vi "VisionMeat.vi"() -> ()   [LabVIEW 2011]
uses:
  <vilib>/vision/NI_Vision_Development_Module.lvlib
  Global 1.vi
panel:
  in  "Camera Type":enum16{"206", "1011"}(ring)
  in  "Score Limits":T1={"Rect Coverage"=76.0, "Aspect Ratio"=70.0, "X Edge Strength"=40.0, "Y Edge Strength"=60.0}
  in  "Area Size Limit":i32=444
  in  "Particle Count Limit":i32=10
  out "Target Info":T2(array[cluster])
  in  "Processing":enum32{"Color", "Intensity", "Intensity Open"}(tab)
  in  "Luminance":i32=255
  in  "Saturation":i32=255
  in  "Hue":i32(knob)=65 scale=0.0..255.0
  in  "Margins":cluster{"Hue":i32, "Sat":i32, "Lum":i32}={"Hue"=9, "Sat"=40, "Lum"=19} {"Sat" scale=0.0..40.0; "Lum" scale=0.0..40.0; "Hue" scale=0.0..40.0}
  in  "Range":cluster{"Lower value":sgl, "Upper value":sgl}={"Lower value"=150.0, "Upper value"=255.0} {"Lower value" scale=0.0..255.0; "Upper value" scale=0.0..255.0}
  in  "Range 2":cluster{"Lower value":sgl, "Upper value":sgl}={"Lower value"=150.0, "Upper value"=255.0} {"Lower value" scale=0.0..255.0; "Upper value" scale=0.0..255.0}
  in  "Annotate":bool=TRUE
  out "Original Image":T3(plugin-control)
  out "Processed Image":T3(plugin-control)
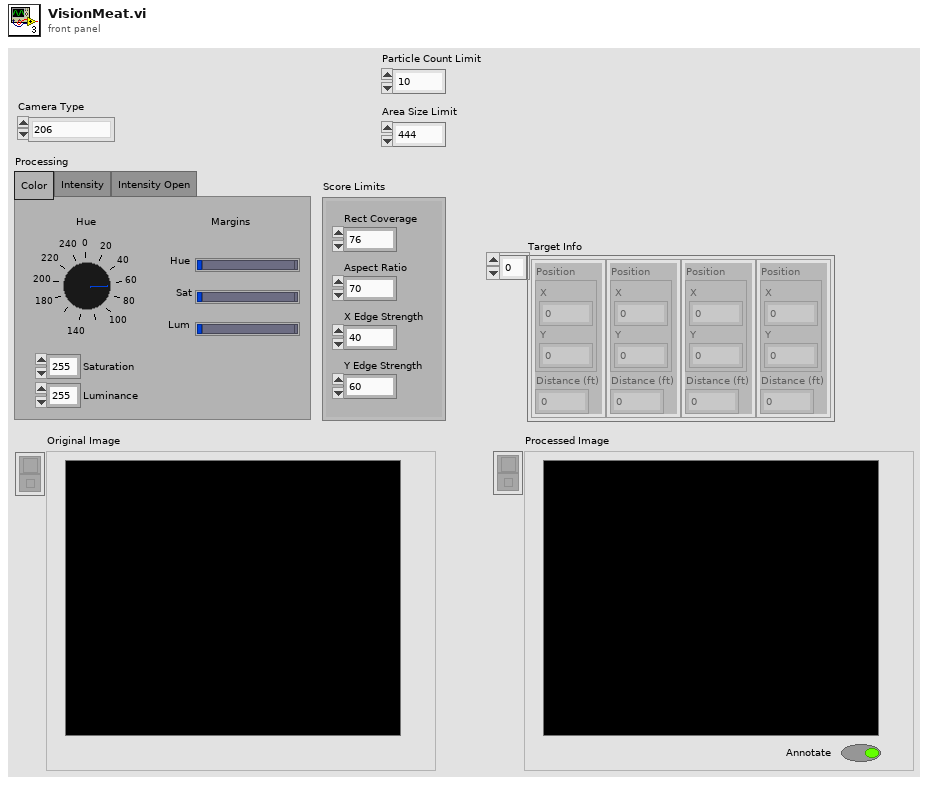
[diagram p1: front panel]
types:
  T1 = cluster{"Rect Coverage":dbl, "Aspect Ratio":dbl, "X Edge Strength":dbl, "Y Edge Strength":dbl}
  T2 = cluster{"Position":cluster{"X":dbl, "Y":dbl}, "Distance (ft)":dbl}[]
  T3 = typedef "IMAQ Image.ctl" = refnum<image>
  T4 = enum32{"AutoM", "Close", "Dilate", "Erode", "Gradient", "Gradient out", "Gradient in", "Hit miss", "Open", "PClose", "POpen", "Thick", "Thin"}
  T5 = cluster{cluster{"Left":dbl, "Top":dbl, "Right":dbl, "Bottom":dbl}, dbl[]}[]
  T6 = cluster{"Left":dbl, "Top":dbl, "Right":dbl, "Bottom":dbl}
  T7 = cluster{"Target Center (-1 to 1)":cluster{"X":dbl, "Y":dbl}, "Distance (ft)":dbl}
  T8 = cluster{"Target Center (-1 to 1)":cluster{"X":dbl, "Y":dbl}, "Distance (ft)":dbl}[]
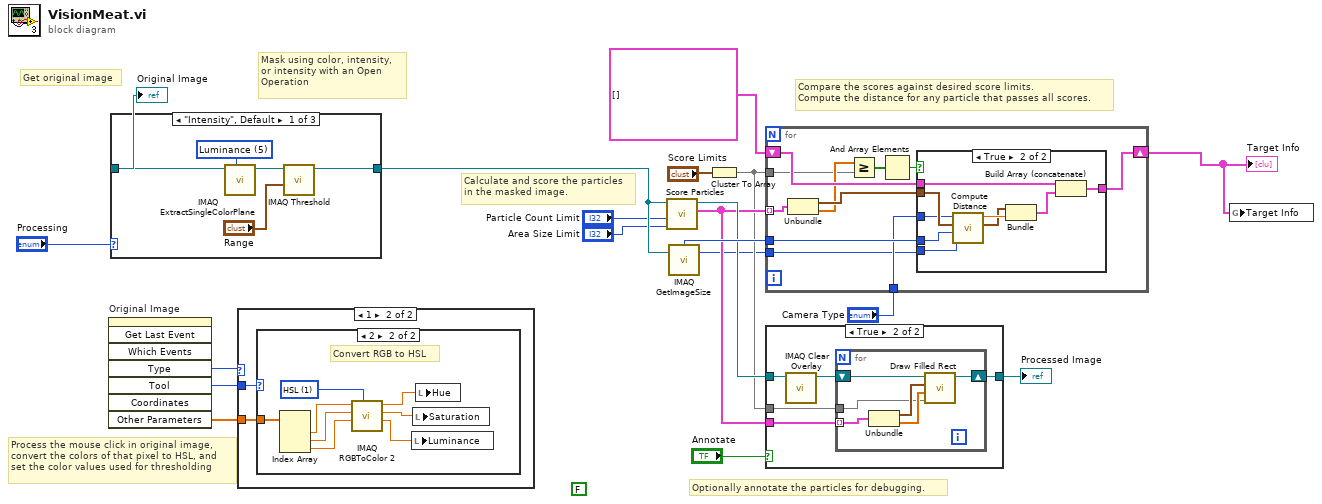
[diagram p0: block diagram]
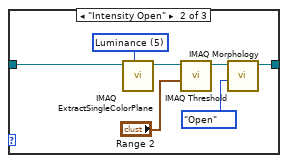
[diagram p3: hidden frame]
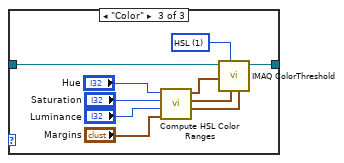
[diagram p4: hidden frame]
diagram:
  (unwired) FALSE
  # "Optionally annotate the particles for debugging."
  # "Compare the scores against desired score limits.\nCompute the distance for any particle that passes all scores."
  # "Process the mouse click in original image,\nconvert the colors of that pixel to HSL, and\nset the color values used for thresholding"
  # "Calculate and score the particles\nin the masked image."
  # "Mask using color, intensity,\nor intensity with an Open\nOperation"
  # "Get original image"
  n1 = invoke on="Original Image" class="ImageControl" method="Get Last Event"() -> ("Type"=w16:i32, "Tool"=w17:i32, "Other Parameters"=w18:sgl[])  [unwired: 8 in, 5 out]
  n2 = case shown="\"Intensity\", Default" "Processing" {
    tunnel: "Original Image" -> [w24 w31 w41]
    tunnel: [w21 w26 w40] -> w7
    frame "Intensity", Default {
      w20 = 5 items=["Red", "Green", "Blue", "Hue", "Saturation", "Luminance", "Value", "Intensity"] ("Color Plane")
      n3 = call "IMAQ ExtractSingleColorPlane"("Color Plane"=w20, "Image Src"=w24) -> ("Image Dst Out"=w23:T3)  [unwired: 2 in, 7 out]
      n4 = call "IMAQ Threshold"("Range"="Range", "Image Src"=w23) -> ("Image Dst Out"=w21:T3)  [unwired: 4 in, 5 out]
    }
    frame "Intensity Open" {
      w25 = 5 items=["Red", "Green", "Blue", "Hue", "Saturation", "Luminance", "Value", "Intensity"] ("Color Plane")
      n5 = call "IMAQ ExtractSingleColorPlane"("Color Plane"=w25, "Image Src"=w31) -> ("Image Dst Out"=w30:T3)  [unwired: 2 in, 7 out]
      n6 = call "IMAQ Threshold"("Range"="Range 2", "Image Src"=w30) -> ("Image Dst Out"=w27:T3)  [unwired: 4 in, 5 out]
      n7 = call "IMAQ Morphology"("Operation"=T4."Open", "Image Src"=w27) -> ("Image Dst Out"=w26:T3)  [unwired: 8 in, 1 out]
    }
    frame "Color" {
      w39 = u16 1 items=["RGB", "HSL", "HSV", "HSI"] ("Color Mode")
      n8 = call "Compute HSL Color Ranges.vi"("Margins"="Margins", "Luminance"="Luminance", "Saturation"="Saturation", "Hue"="Hue") -> ("Lum Range"=w36:cluster{i32, i32}, "Sat Range"=w37:cluster{i32, i32}, "Hue Range"=w38:cluster{i32, i32})  [unwired: 5 in]
      n9 = call "IMAQ ColorThreshold"("Blue or Luma or Val or Inten Range"=w36, "Green or Sat Range"=w37, "Color Mode"=w39, "Red or Hue Range"=w38, "Image Src"=w41) -> ("Image Dst Out"=w40:T3)  [unwired: 5 in, 1 out]
    }
  }
  n10 = case shown="1" w16 {
    tunnel: w17 -> [_ w43]
    tunnel: w18 -> [_ w42]
    frame 0, Default {
    }
    frame 1 {
      n11 = case shown="2" w43 {
        tunnel: w42 -> [_ w51]
        frame Default {
        }
        frame 2 {
          w50 = u16 1 items=["RGB", "HSL", "HSV", "HSI", "CIE L*a*b*", "CIE XYZ"] ("Color Mode")
          # "Convert RGB to HSL"
          n12 = Index Array(array=w51) -> (element #1=w49:sgl, element #2=w47:sgl, element #3=w45:sgl)  [unwired: 3 in]
          n13 = call "IMAQ RGBToColor 2"("Color Mode"=w50, "Blue value"=w45, "Green value"=w47, "Red value"=w49) -> ("Blue or Luma or Val or Inten or Z or b*value"=w44:dbl, "Green or Sat or Y or a* value"=w46:dbl, "Red or Hue or X or L* value"=w48:dbl)  [unwired: 4 in, 1 out]
          n14 = local write "Luminance"(w44) -> ()
          n15 = local write "Saturation"(w46) -> ()
          n16 = local write "Hue"(w48) -> ()
        }
      }
    }
  }
  n17 = call "Score Particles.vi"("Area Size Limit"="Area Size Limit", "Particle Count Limit"="Particle Count Limit", "Image Refnum in"=w7) -> ("Scored Particle Info"=w10:T5, "Image Refnum out"=w14:T3)  [unwired: 7 in]
  n18 = call "IMAQ GetImageSize"("Image"=w7) -> ("Y Resolution"=w3:i32, "X Resolution"=w15:i32)  [unwired: 3 in, 1 out]
  n19 = Cluster To Array(cluster="Score Limits") -> (array=w8:dbl[])
  n20 = for {
    shift-right: [w61] -> w1
    shift-left: T2 [] -> [w62]
    tunnel: w15 -> [w60]
    tunnel: w10 -> [w58] mode=indexing
    tunnel: w8 -> [w53]
    tunnel: "Camera Type" -> [w57]
    tunnel: w3 -> [w52]
    n21 = Unbundle(w58) -> (w59:T6, w54:dbl[])
    n22 = Greater Or Equal?(x=w54, y=w53) -> (x >= y?=w56:bool[])
    n23 = And Array Elements(Boolean array=w56) -> (logical AND=w55:bool)
    n24 = case shown="True" w55 {
      tunnel: w62 -> [w63 w72]
      tunnel: [w63 w71] -> w61
      tunnel: w59 -> [_ w67]
      tunnel: w60 -> [_ w69]
      tunnel: w57 -> [_ w66]
      tunnel: w52 -> [_ w64]
      frame False {
      }
      frame True {
        n25 = call "Compute Distance.vi"("Y Image Resolution"=w64, "X Image Resolution"=w69, "Bounding Box"=w67, "Camera Type"=w66) -> ("Target Center (-1 to 1)"=w65:cluster{"X":dbl, "Y":dbl}, "Distance (ft)"=w68:dbl)  [unwired: 6 in]
        n26 = Bundle("Target Center (-1 to 1)"=w65, "Distance (ft)"=w68) -> (w70:T7)  [unwired: 1 in]
        n27 = Build Array (concatenate)(w72, w70) -> (w71:T8)
      }
    }
  }
  "Target Info" <- w1
  n28 = case shown="True" "Annotate" {
    tunnel: w14 -> [w73 w78]
    tunnel: [w73 w77] -> w11
    tunnel: w10 -> [_ w75]
    tunnel: w8 -> [_ w74]
    frame False {
    }
    frame True {
      n29 = call "IMAQ Clear Overlay"("Image"=w78) -> ("Image Out"=w76:T3)  [unwired: 2 in, 8 out]
      n30 = for {
        shift-right: [w83] -> w77
        shift-left: w76 -> [w84]
        tunnel: w75 -> [w80] mode=indexing
        tunnel: w74 -> [w79]
        n31 = Unbundle(w80) -> (w81:T6, w82:dbl[])
        n32 = call "Draw Filled Rect.vi"("Limits"=w79, "Scores"=w82, "Bounding Box"=w81, "image in"=w84) -> ("image out"=w83:T3)  [unwired: 7 in]
      }
    }
  }
  "Processed Image" <- w11
  n33 = global write "Global 1.vi" "Target Info"(w1) -> ()
